vi "Config HW Extract.vi"(6 "Send Cmd Timout(ms)":u32=300, 7 "CANcoderRef":T1, 8 "Error":errorcluster, 9 "CAN.Bus":string, 10 "HW Config":T2={"LiftHW Ver"=0, "CAN"={"ID Primary"=0, "Bus"="", "ID Follower"=0}, "Output"={"Type"=enum."Counter-Clockwise", "Neutral"=enum."Override to Coast", "Max"={"FWD"=1.0, "REV"=-1.0}, "Min"={"FWD"=0.0, "REV"=0.0}, "OL Ramp Rate (S)"=0.0, "Dead Band"=0.0}, "CLUp"={"Gains"={"P"=1.0, "I"=0.01, "D"=0.0, "F"=0.0}, "Error Allowed"={"High"=0.0, "Low"=0.0}, "I Zone"={"High"=10000.0, "Low"=-1000.0}, "Max Out"={"FWD"=1.0, "REV"=-1.0}, "Max I Accu"={"High"=10.0, "Low"=-10.0}, "CL Ramp Rate (S)"=0.0}, "MM"={"Cruise Velocity"=5000, "Acceleration"=5000}, "TravelLimits"={"Hard"={"FWD Switch Normal"=enum."Normally Open", "FWD On will Zero Encoder "=FALSE, "REV Switch Normal"=enum."Normally Open", "REV On will Zero Encoder "=FALSE}, "Soft"={"FWD"={"Enable"=FALSE, "Counts"=0}, "REV"={"Enable"=FALSE, "Counts"=0}}}, "Cancoder"={"ID"=0, "CW(t) CCW(f)"=TRUE, "Zero Offset"=0.0}, "CLDown"={"Gains"={"P"=1.0, "I"=0.01, "D"=0.0, "F"=0.0}, "Error Allowed"={"High"=0.0, "Low"=0.0}, "I Zone"={"High"=10000.0, "Low"=-1000.0}, "Max Out"={"FWD"=1.0, "REV"=-1.0}, "Max I Accu"={"High"=10.0, "Low"=-10.0}, "CL Ramp Rate (S)"=0.0}, "CurrentLimit"={"Enable"=FALSE, "Current Limit"=0.0, "Threshold Current"=0.0, "Threshold Time"=0.0}} {"CLDown"."Max I Accu"."Low" format="%#.8f"; "CLDown"."Max I Accu"."High" format="%#.8f"; "CLDown"."Gains"."F" format="%#.8f"; "CLDown"."Gains"."D" format="%#.8f"; "CLDown"."Gains"."I" format="%#.8f"; "CLDown"."Gains"."P" format="%#.8f"; "CLDown"."Error Allowed"."Low" format="%#.8f"; "CLDown"."Error Allowed"."High" format="%#.8f"; "CLDown"."I Zone"."Low" format="%#.8f"; "CLDown"."I Zone"."High" format="%#.8f"; "CLDown"."Max Out"."REV" format="%.2f"; "CLDown"."Max Out"."FWD" format="%.2f"; "TravelLimits"."Soft"."REV"."Counts" format="%#.0f"; "TravelLimits"."Soft"."FWD"."Counts" format="%#.0f"; "Output"."Min"."REV" format="%.2f"; "Output"."Min"."FWD" format="%.2f"; "Output"."Max"."REV" format="%.2f"; "Output"."Max"."FWD" format="%.2f"; "CLUp"."Max I Accu"."Low" format="%#.8f"; "CLUp"."Max I Accu"."High" format="%#.8f"; "CLUp"."Gains"."F" format="%#.8f"; "CLUp"."Gains"."D" format="%#.8f"; "CLUp"."Gains"."I" format="%#.8f"; "CLUp"."Gains"."P" format="%#.8f"; "CLUp"."Error Allowed"."Low" format="%#.8f"; "CLUp"."Error Allowed"."High" format="%#.8f"; "CLUp"."I Zone"."Low" format="%#.8f"; "CLUp"."I Zone"."High" format="%#.8f"; "CLUp"."Max Out"."REV" format="%.2f"; "CLUp"."Max Out"."FWD" format="%.2f"}, 11 "DevRef":T19={"DeviceStatus"={"status"=FALSE, "code"=0, "source"=""}, "Type"=enum."PWM", "PWM"={"PWM Channel"=enum."Invalid", "DeadBand"={"Name"="", "maxPositivePwm"=0, "minPositivePwm"=0, "centerPwm"=0, "maxNegativePwm"=0, "minNegativePwm"=0, "angularRange"=0}}, "CAN"={"Device Number"=0, "SetOutput VI Ref"=variant, "GetOutput VI Ref"=variant, "Enable VI Ref"=variant, "Disable VI Ref"=variant, "Data"=variant}, "Invert"=FALSE, "DIO PWM"={"PWM \"Enable\" Channel"=enum."Invalid", "DIOChannel"=enum."Invalid", "PWM Rate"=0.0}}) -> (0 "Error Out":errorcluster, 2 "HW Config Data Out":T2={"LiftHW Ver"=0, "CAN"={"ID Primary"=0, "Bus"="", "ID Follower"=0}, "Output"={"Type"=enum."Counter-Clockwise", "Neutral"=enum."Override to Coast", "Max"={"FWD"=1.0, "REV"=-1.0}, "Min"={"FWD"=0.0, "REV"=0.0}, "OL Ramp Rate (S)"=0.0, "Dead Band"=0.0}, "CLUp"={"Gains"={"P"=1.0, "I"=0.01, "D"=0.0, "F"=0.0}, "Error Allowed"={"High"=0.0, "Low"=0.0}, "I Zone"={"High"=10000.0, "Low"=-1000.0}, "Max Out"={"FWD"=1.0, "REV"=-1.0}, "Max I Accu"={"High"=10.0, "Low"=-10.0}, "CL Ramp Rate (S)"=0.0}, "MM"={"Cruise Velocity"=5000, "Acceleration"=5000}, "TravelLimits"={"Hard"={"FWD Switch Normal"=enum."Normally Open", "FWD On will Zero Encoder "=FALSE, "REV Switch Normal"=enum."Normally Open", "REV On will Zero Encoder "=FALSE}, "Soft"={"FWD"={"Enable"=FALSE, "Counts"=0}, "REV"={"Enable"=FALSE, "Counts"=0}}}, "Cancoder"={"ID"=0, "CW(t) CCW(f)"=TRUE, "Zero Offset"=0.0}, "CLDown"={"Gains"={"P"=1.0, "I"=0.01, "D"=0.0, "F"=0.0}, "Error Allowed"={"High"=0.0, "Low"=0.0}, "I Zone"={"High"=10000.0, "Low"=-1000.0}, "Max Out"={"FWD"=1.0, "REV"=-1.0}, "Max I Accu"={"High"=10.0, "Low"=-10.0}, "CL Ramp Rate (S)"=0.0}, "CurrentLimit"={"Enable"=FALSE, "Current Limit"=0.0, "Threshold Current"=0.0, "Threshold Time"=0.0}} {"CLDown"."Max I Accu"."Low" format="%#.8f"; "CLDown"."Max I Accu"."High" format="%#.8f"; "CLDown"."Gains"."F" format="%#.8f"; "CLDown"."Gains"."D" format="%#.8f"; "CLDown"."Gains"."I" format="%#.8f"; "CLDown"."Gains"."P" format="%#.8f"; "CLDown"."Error Allowed"."Low" format="%#.8f"; "CLDown"."Error Allowed"."High" format="%#.8f"; "CLDown"."I Zone"."Low" format="%#.8f"; "CLDown"."I Zone"."High" format="%#.8f"; "CLDown"."Max Out"."REV" format="%.2f"; "CLDown"."Max Out"."FWD" format="%.2f"; "TravelLimits"."Soft"."REV"."Counts" format="%#.0f"; "TravelLimits"."Soft"."FWD"."Counts" format="%#.0f"; "Output"."Min"."REV" format="%.2f"; "Output"."Min"."FWD" format="%.2f"; "Output"."Max"."REV" format="%.2f"; "Output"."Max"."FWD" format="%.2f"; "CLUp"."Max I Accu"."Low" format="%#.8f"; "CLUp"."Max I Accu"."High" format="%#.8f"; "CLUp"."Gains"."F" format="%#.8f"; "CLUp"."Gains"."D" format="%#.8f"; "CLUp"."Gains"."I" format="%#.8f"; "CLUp"."Gains"."P" format="%#.8f"; "CLUp"."Error Allowed"."Low" format="%#.8f"; "CLUp"."Error Allowed"."High" format="%#.8f"; "CLUp"."I Zone"."Low" format="%#.8f"; "CLUp"."I Zone"."High" format="%#.8f"; "CLUp"."Max Out"."REV" format="%.2f"; "CLUp"."Max Out"."FWD" format="%.2f"}, 3 "DevRef Out":T19, 5 "CANcoderRef Out":T1)   [LabVIEW 2020, in "Lift_ACT.lvlib"]
uses:
  Lift_ACT.lvlib
  <vilib>/Rock Robotics/WPI/MotorControl/WPI_MotorControlDeviceRef.ctl
  <vilib>/Rock Robotics/WPI/MotorControl/WPI_MotorControlType.ctl
  <vilib>/Rock Robotics/SystemInterfaces/DIO/FPGA_DIOPWMChannel.ctl
  <vilib>/Rock Robotics/WPI/PWM/WPI_PWMDeadband.ctl
  <vilib>/Rock Robotics/SystemInterfaces/DIO/FPGA_DIOChannel.ctl
  Shared Code/TypeDefs/Cluster_Lift_Config HW Values.ctl
  Shared Code/TypeDefs/Cluser_CAN Follower Data.ctl
  Shared Code/TypeDefs/Cluster_Config Motor Output.ctl
  <vilib>/Rock Robotics/WPI/ThirdParty/Phoenix-LabVIEW/Motor Controller/Controls/CTRE_Phoenix_MotorControl_TalonFXInvertType.ctl
  <vilib>/Rock Robotics/WPI/ThirdParty/Phoenix-LabVIEW/Motor Controller/Controls/CTRE_Phoenix_MotorControl_NeutralMode.ctl
  Shared Code/TypeDefs/Cluster_FWD  REV Values.ctl
  Shared Code/TypeDefs/Cluster_PID Config.ctl
  Shared Code/TypeDefs/Cluster_PID Gains.ctl
  Shared Code/TypeDefs/Cluster_High-Low.ctl
  Shared Code/TypeDefs/Cluster_Motion Magic Parameters.ctl
  Shared Code/TypeDefs/Cluser_Limit Travel Config.ctl
  Shared Code/TypeDefs/Cluser_Hard Limits.ctl
  <vilib>/Rock Robotics/WPI/ThirdParty/Phoenix-LabVIEW/Motor Controller/Controls/CTRE_Phoenix_MotorControl_LimitSwitchNormal.ctl
  Shared Code/TypeDefs/Cluser_Config_Soft Limits.ctl
  Shared Code/TypeDefs/Cluser_Enable-Value I32.ctl
  Shared Code/TypeDefs/Cluster_Config_Cancoder Data.ctl
  Shared Code/TypeDefs/Cluser_Config_Current Limits.ctl
  <vilib>/Rock Robotics/WPI/ThirdParty/Phoenix-LabVIEW/CANCoder/Controls/CTRE_Phoenix_CANcoder_DeviceRef.ctl
  Shared Code/TypeDefs/Cluser_CAN Data.ctl
panel:
  # "Tune Output\nto 1023 Max"
  # "Tune Output\nto 1023 Max"
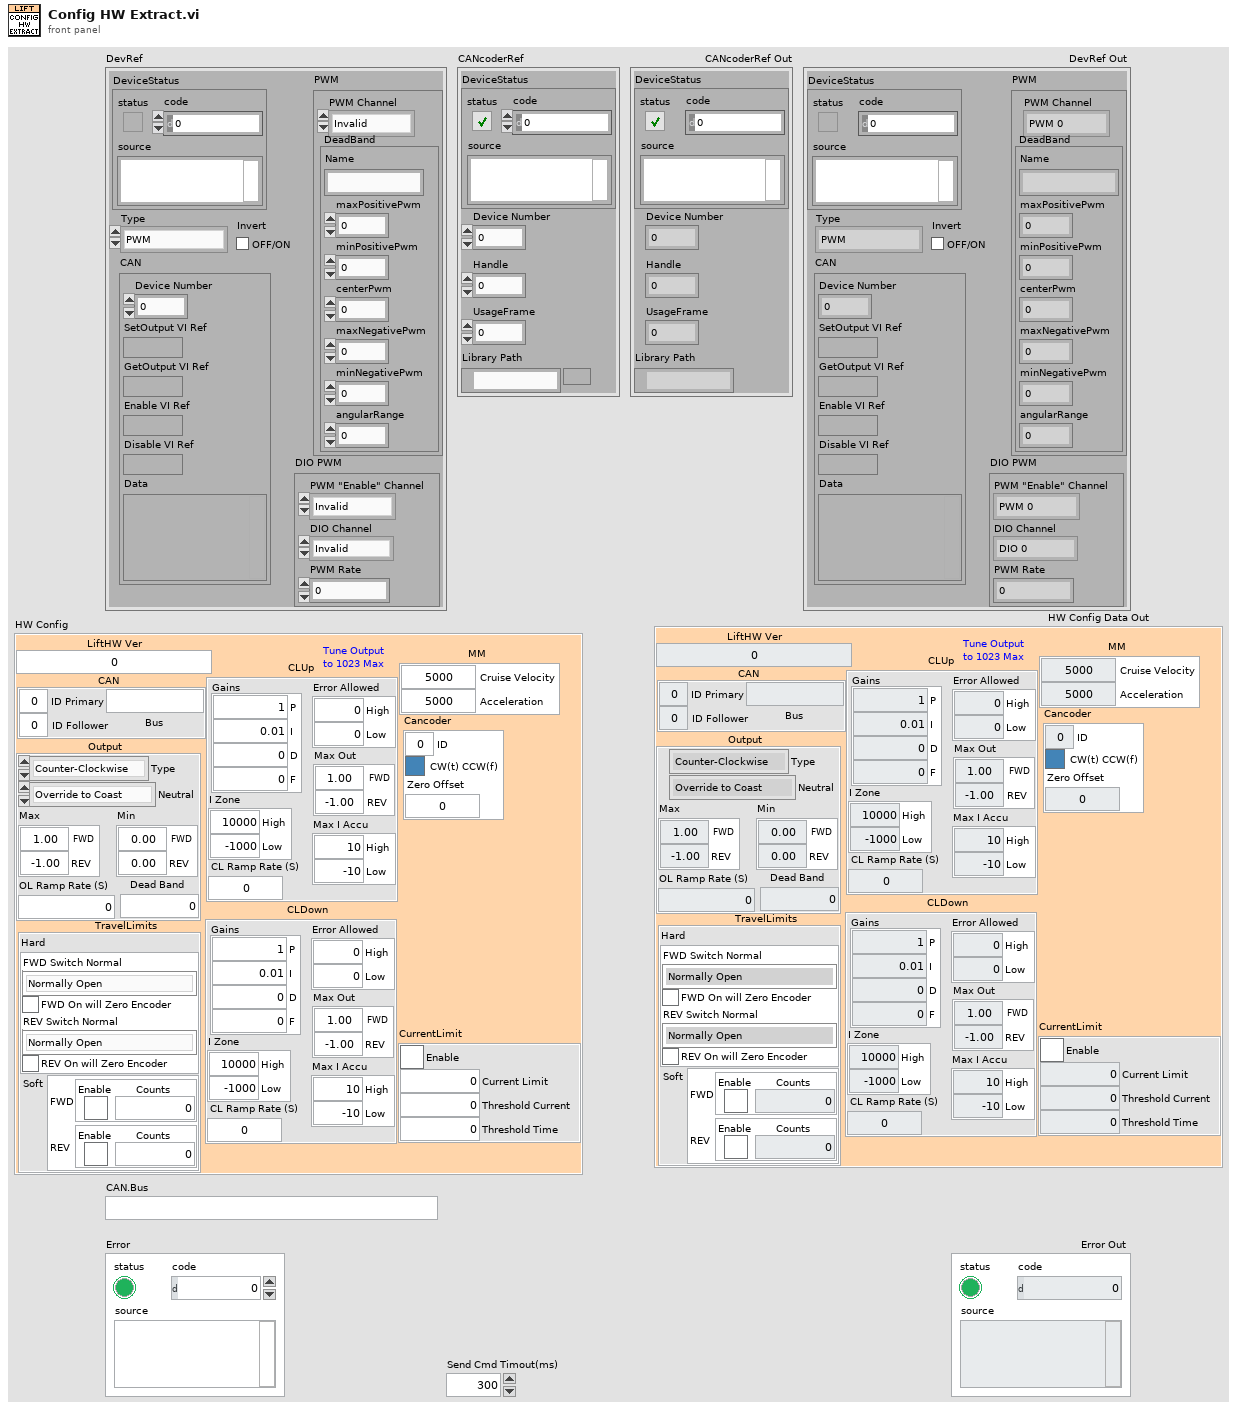
[diagram p1: front panel]
types:
  T1 = typedef "CTRE_Phoenix_CANcoder_DeviceRef.ctl" = cluster{"DeviceStatus":errorcluster, "Device Number":u8, "Handle":u64, "UsageFrame":u32, "Library Path":path}
  T2 = typedef "Cluster_Lift_Config HW Values.ctl" = cluster{"LiftHW Ver":u64, "CAN":T3, "Output":T4, "CLUp":T8, "MM":T11, "TravelLimits":T12, "Cancoder":T17, "CLDown":T8, "CurrentLimit":T18}
  T3 = typedef "Cluser_CAN Follower Data.ctl" = cluster{"ID Primary":u8, "Bus":string, "ID Follower":u8}
  T4 = typedef "Cluster_Config Motor Output.ctl" = cluster{"Type":T5, "Neutral":T6, "Max":T7, "Min":T7, "OL Ramp Rate (S)":dbl, "Dead Band":dbl}
  T5 = typedef "CTRE_Phoenix_MotorControl_TalonFXInvertType.ctl" = enum16{"Counter-Clockwise", "Clockwise"}
  T6 = typedef "CTRE_Phoenix_MotorControl_NeutralMode.ctl" = enum8{"EEPROMSetting", "Override to Coast", "Override to Brake"}
  T7 = typedef "Cluster_FWD  REV Values.ctl" = cluster{"FWD":dbl, "REV":dbl}
  T8 = typedef "Cluster_PID Config.ctl" = cluster{"Gains":T9, "Error Allowed":T10, "I Zone":T10, "Max Out":T7, "Max I Accu":T10, "CL Ramp Rate (S)":dbl}
  T9 = typedef "Cluster_PID Gains.ctl" = cluster{"P":dbl, "I":dbl, "D":dbl, "F":dbl}
  T10 = typedef "Cluster_High-Low.ctl" = cluster{"High":dbl, "Low":dbl}
  T11 = typedef "Cluster_Motion Magic Parameters.ctl" = cluster{"Cruise Velocity":i32, "Acceleration":i32}
  T12 = typedef "Cluser_Limit Travel Config.ctl" = cluster{"Hard":T13, "Soft":T15}
  T13 = typedef "Cluser_Hard Limits.ctl" = cluster{"FWD Switch Normal":T14, "FWD On will Zero Encoder ":bool, "REV Switch Normal":T14, "REV On will Zero Encoder ":bool}
  T14 = typedef "CTRE_Phoenix_MotorControl_LimitSwitchNormal.ctl" = enum16{"Normally Open", "Normally Closed", "Disabled"}
  T15 = typedef "Cluser_Config_Soft Limits.ctl" = cluster{"FWD":T16, "REV":T16}
  T16 = typedef "Cluser_Enable-Value I32.ctl" = cluster{"Enable":bool, "Counts":i32}
  T17 = typedef "Cluster_Config_Cancoder Data.ctl" = cluster{"ID":u8, "CW(t) CCW(f)":bool, "Zero Offset":dbl}
  T18 = typedef "Cluser_Config_Current Limits.ctl" = cluster{"Enable":bool, "Current Limit":dbl, "Threshold Current":dbl, "Threshold Time":dbl}
  T19 = typedef "WPI_MotorControlDeviceRef.ctl" = cluster{"DeviceStatus":errorcluster, "Type":T20, "PWM":cluster{"PWM Channel":T21, "DeadBand":T22}, "CAN":cluster{"Device Number":u8, "SetOutput VI Ref":variant, "GetOutput VI Ref":variant, "Enable VI Ref":variant, "Disable VI Ref":variant, "Data":variant}, "Invert":bool, "DIO PWM":cluster{"PWM \"Enable\" Channel":T21, "DIOChannel":T23, "PWM Rate":dbl}}
  T20 = typedef "WPI_MotorControlType.ctl" = enum16{"PWM", "CAN", "DIO PWM"}
  T21 = typedef "FPGA_DIOPWMChannel.ctl" = enum8{"PWM 0", "PWM 1", "PWM 2", "PWM 3", "PWM 4", "PWM 5", "PWM 6", "PWM 7", "PWM 8", "PWM 9", "PWM MXP 0", "PWM MXP 1", "PWM MXP 2", "PWM MXP 3", "PWM MXP 4", "PWM MXP 5", "PWM MXP 6", "PWM MXP 7", "PWM MXP 8", "PWM MXP 9", "Invalid"}
  T22 = typedef "WPI_PWMDeadband.ctl" = cluster{"Name":string, "maxPositivePwm":i32, "minPositivePwm":i32, "centerPwm":i32, "maxNegativePwm":i32, "minNegativePwm":i32, "angularRange":u16}
  T23 = typedef "FPGA_DIOChannel.ctl" = enum8{"DIO 0", "DIO 1", "DIO 2", "DIO 3", "DIO 4", "DIO 5", "DIO 6", "DIO 7", "DIO 8", "DIO 9", "DIO MXP 0", "DIO MXP 1", "DIO MXP 2", "DIO MXP 3", "DIO MXP 4", "DIO MXP 5", "DIO MXP 6", "DIO MXP 7", "DIO MXP 8", "DIO MXP 9", "DIO MXP 10", "DIO MXP 11", "DIO MXP 12", "DIO MXP 13", "DIO MXP 14", "DIO MXP 15", "SPI Port CS1", "SPI Port CS2", "SPI Port CS3", "SPI Port MISO", "SPI Port MOSI", "Invalid"}
  T24 = typedef "Cluser_CAN Data.ctl" = cluster{"ID":u8, "Bus":string}
  T25 = typedef "CTRE_Phoenix_CANcoder_Configurables.ctl" = cluster{"Sensor Initialization Strategy":T26, "Absolute Sensor Range":T27, "Velocity Measurement Period":T28, "Velocity Measurement Window":i32, "Magnet Offset (Degrees)":dbl, "Sensor Direction":bool, "Sensor Coefficient":dbl, "Unit String":string, "Sensor Time Base":T29}
  T26 = typedef "CTRE_Phoenix_CANcoder_SensorInitializationStrategy.ctl" = enum16{"Boot To Zero", "Boot To Absolute Position"}
  T27 = typedef "CTRE_Phoenix_CANcoder_AbsoluteSensorRange.ctl" = enum16{"Unsigned [0 to 360)", "Signed [-180 to +180)"}
  T28 = typedef "CTRE_Phoenix_MotorControl_VelocityMeasurementPeriod.ctl" = u16
  T29 = typedef "CTRE_Phoenix_CANcoder_SensorTimeBase.ctl" = enum16{"Per100Ms_Legacy", "PerSecond", "PerMinute"}
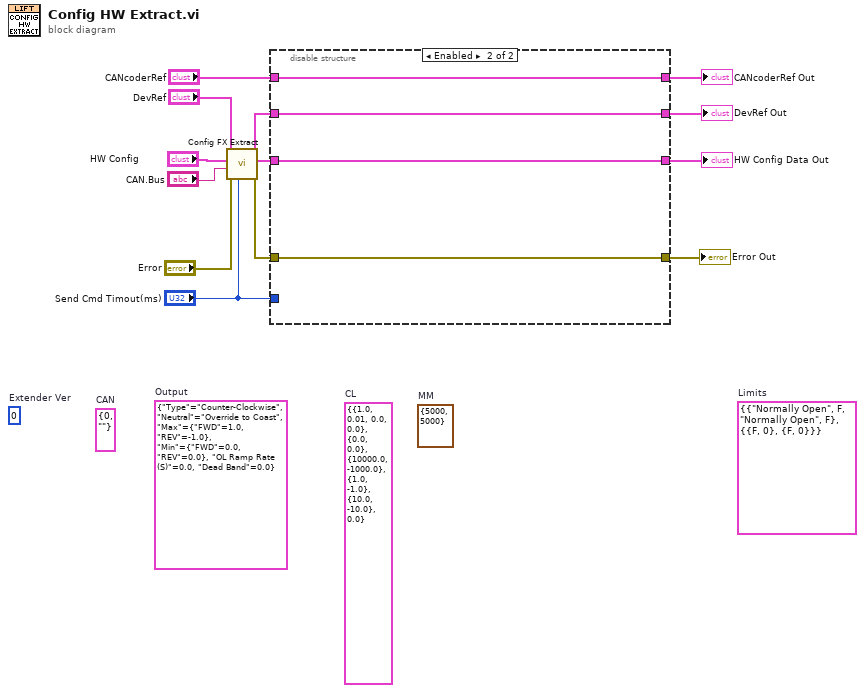
[diagram p0: block diagram]
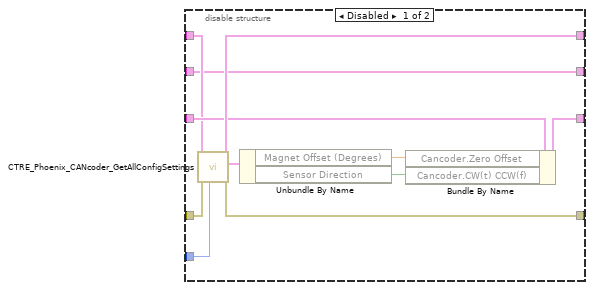
[diagram p2: hidden frame]
diagram:
  (unwired) T12 {"Hard"={"FWD Switch Normal"=enum."Normally Open", "FWD On will Zero Encoder "=FALSE, "REV Switch Normal"=enum."Normally Open", "REV On will Zero Encoder "=FALSE}, "Soft"={"FWD"={"Enable"=FALSE, "Counts"=0}, "REV"={"Enable"=FALSE, "Counts"=0}}}  # Limits
  (unwired) T11 {"Cruise Velocity"=5000, "Acceleration"=5000}  # MM
  (unwired) T4 {"Type"=enum."Counter-Clockwise", "Neutral"=enum."Override to Coast", "Max"={"FWD"=1.0, "REV"=-1.0}, "Min"={"FWD"=0.0, "REV"=0.0}, "OL Ramp Rate (S)"=0.0, "Dead Band"=0.0}  # Output
  (unwired) u64 0  # Extender Ver
  (unwired) T24 {"ID"=0, "Bus"=""}  # CAN
  (unwired) T8 {"Gains"={"P"=1.0, "I"=0.01, "D"=0.0, "F"=0.0}, "Error Allowed"={"High"=0.0, "Low"=0.0}, "I Zone"={"High"=10000.0, "Low"=-1000.0}, "Max Out"={"FWD"=1.0, "REV"=-1.0}, "Max I Accu"={"High"=10.0, "Low"=-10.0}, "CL Ramp Rate (S)"=0.0}  # CL
  n1 = call "Config FX Extract.vi"("Send Cmd Timout(ms)"="Send Cmd Timout(ms)", "Error"="Error", "CAN.Bus"="CAN.Bus", "HW Config"="HW Config", "PhoenixMotorControlDevRef"="DevRef") -> ("Error Out"=w10:errorcluster, "HW Config Data Out"=w12:T2, "Module Azimuth Ref Out"=w2:T19)  [unwired: 4 in]
  n2 = disable-structure shown="Enabled" {
    disable-tunnel: [w24 w28] -> w13
    disable-tunnel: w12 -> [w22 w26]
    disable-tunnel: [w21 w26] -> w11
    disable-tunnel: w10 -> [w18 w25]
    disable-tunnel: "CANcoderRef" -> [w17 w28]
    disable-tunnel: [w16 w25] -> w7
    disable-tunnel: "Send Cmd Timout(ms)" -> [w15 _]
    disable-tunnel: w2 -> [w14 w27]
    disable-tunnel: [w14 w27] -> w1
    frame Disabled {
      n3 = call <vilib>:"CTRE_Phoenix_CANcoder_GetAllConfigSettings.vi"("timeoutMs"=w15, "error in (no error)"=w18, "CTRE_CANcoder_DeviceRef"=w17) -> ("error out"=w16:errorcluster, "CANcoder Configurables"=w23:T25, "CTRE_CANcoder_DeviceRef"=w24:T1)  [unwired: 6 in]
      n4 = Unbundle By Name(w23) -> ("Magnet Offset (Degrees)"=w20:dbl, "Sensor Direction"=w19:bool)
      n5 = Bundle By Name(cluster=w22, "Cancoder.Zero Offset"=w20, "Cancoder.CW(t) CCW(f)"=w19) -> (w21:T2)
    }
    frame Enabled {
    }
  }
  "DevRef Out" <- w1
  "Error Out" <- w7
  "HW Config Data Out" <- w11
  "CANcoderRef Out" <- w13
